vi "BBO.vi"() -> ()   [LabVIEW 2014]
doc: "The myRIO Project template acquires acceleration data from the onboard accelerometer and displays the changes of acceleration values in a waveform chart."
uses:
  <vilib>/vision/driver/NI_Vision_Acquisition_Software.lvlib
  <vilib>/vision/NI_Vision_Development_Module.lvlib
panel:
  in  "배경색ROI밑 자름":dbl=15.0
  in  "위":dbl=60.0
  in  "오른쪽":dbl=60.0
  in  "왼쪽":dbl=40.0
  in  "카메라 X부호":dbl=1.0
  in  "카메라 X":dbl=18.0
  in  "Select Servo 2":string(combo)="Servo 2"
  in  "Threshold Color Mode 3":enum32{"RGB", "HSL"}(radio)=enum."HSL"
  in  "Red or Hue 5":cluster{i32, i32}(slide)={0, 255} scale=0.0..255.0
  in  "Green or Saturation 5":cluster{i32, i32}(slide)={0, 35} scale=0.0..255.0
  in  "Blue or Luminance 5":cluster{i32, i32}(slide)={0, 75} scale=0.0..255.0
  out "볼링핀을찾았는가":bool
  in  "화면전환":bool=TRUE
  out "Image 3":T1(plugin-control)
  in  "공 굴릴 범위":dbl=10.0
  in  "작게 움직이는 범위":dbl=500.0
  in  "탭컨트롤":dbl
  in  "탭 컨트롤":enum32{"볼링핀 0", "녹색핀 1"}(tab)
  in  "Blue or Luminance":cluster{i32, i32}(slide)={90, 255} scale=0.0..255.0
  in  "Green or Saturation":cluster{i32, i32}(slide)={0, 90} scale=0.0..255.0
  in  "Red or Hue":cluster{i32, i32}(slide)={0, 255} scale=0.0..255.0
  in  "Blue or Luminance 3":cluster{i32, i32}(slide)={60, 255} scale=0.0..255.0
  in  "Green or Saturation 3":cluster{i32, i32}(slide)={35, 255} scale=0.0..255.0
  in  "Red or Hue 3":cluster{i32, i32}(slide)={50, 130} scale=0.0..255.0
  in  "좌우모터":i16=25
  in  "Number of Erosion":i32=2
  in  "Threshold Color Mode":enum32{"RGB", "HSL"}(radio)=enum."HSL"
  out "Image 2":T1(plugin-control)
  out "Image":T1(plugin-control)
  in  "Camera Name":refnum<k21>="cam1" caption="IMAQdx Session"
  # "Control Motor"
  # "Read Encoder"
  # "배경색(검은색) 색조"
  # "255"
  # "25"
  # "채도"
  # "HSL : 색조 채도 광도"
  # "35"
  # "광도"
  # "75"
  # "1일때 + 0일때 -"
  # "흰색 : 0/255"
  # "흰색 : 0~90"
  # "흰색 : 90~255"
  # "녹색 : 50/130"
  # "녹색 : 35/255"
  # "녹색 : 60/255"
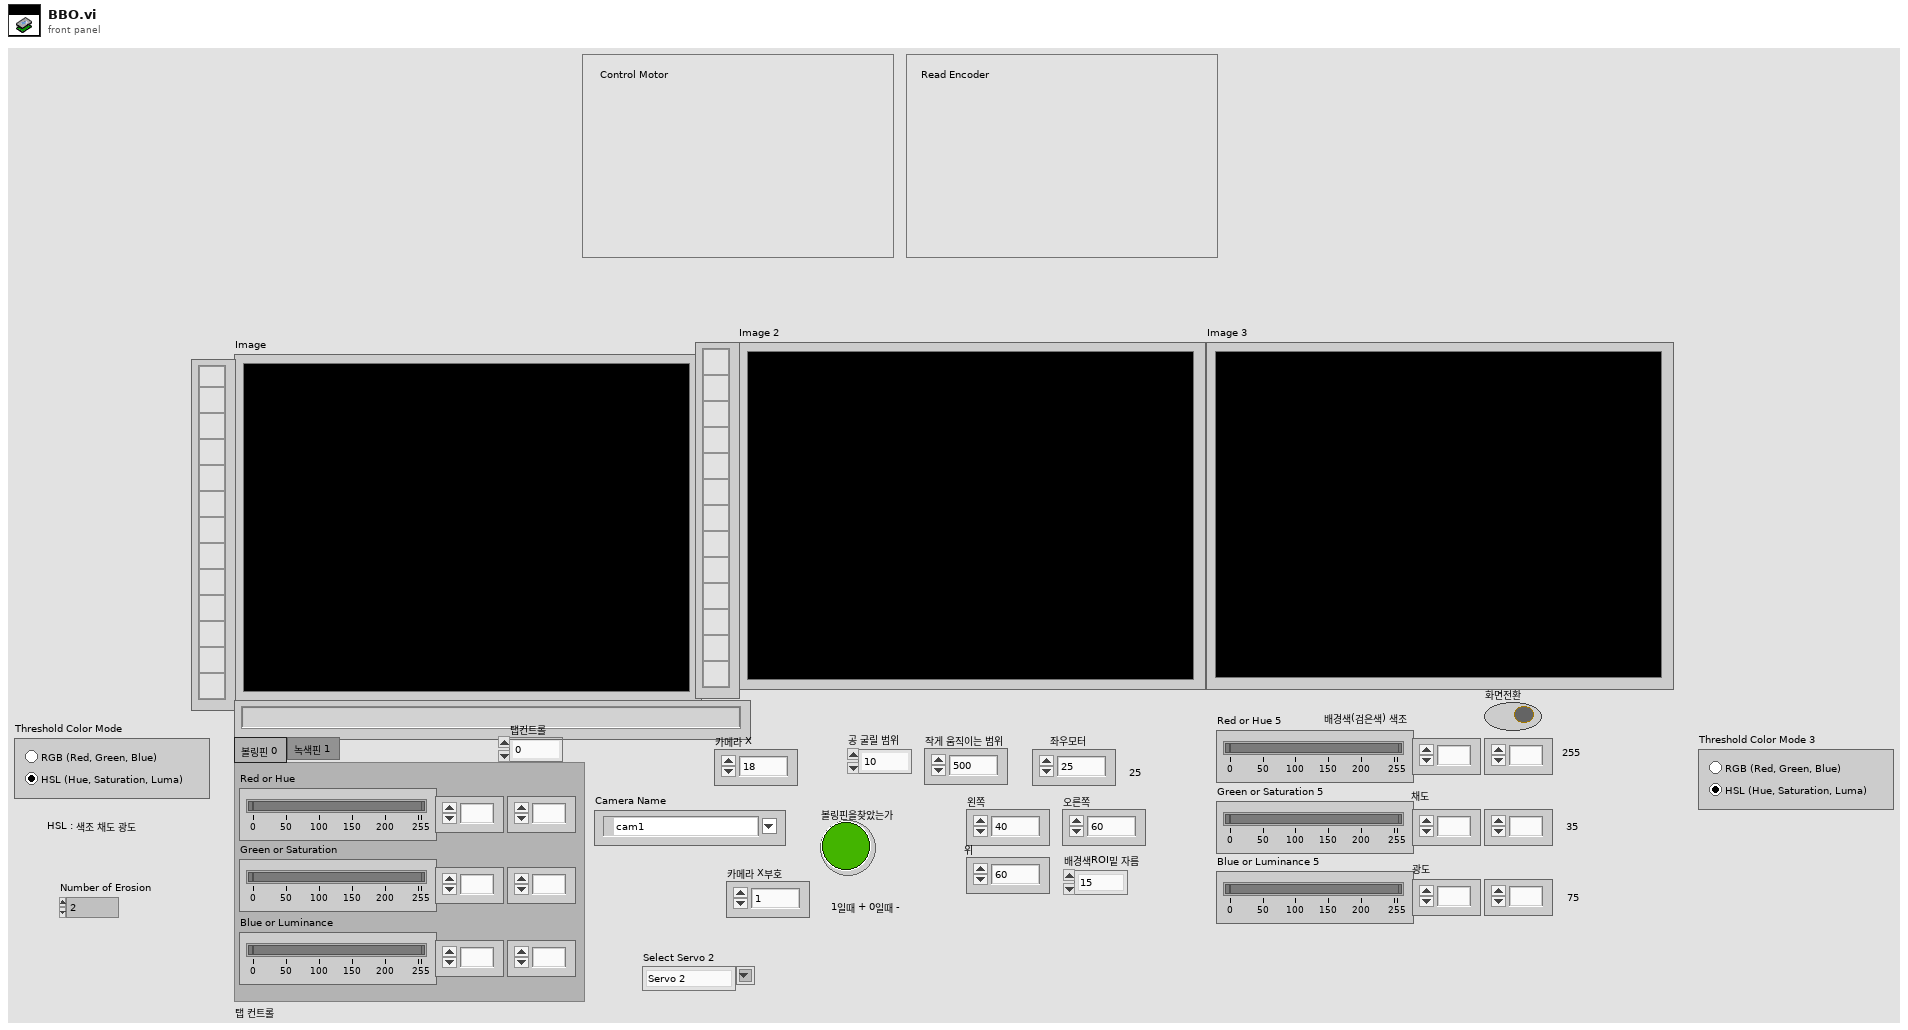
[diagram p1: front panel]
types:
  T1 = typedef "IMAQ Image.ctl" = refnum<image>
  T2 = typedef "IMAQ Rectangle" = cluster{"Left":i32, "Top":i32, "Right":i32, "Bottom":i32, "Rotation":dbl}
  T3 = typedef "Image Type" = u32
  T4 = typedef "IMAQdx.ctl" = refnum<k21>
  T5 = cluster{"Area":dbl, "Number of Holes":dbl, "Bounding Rect":cluster{"Left":dbl, "Top":dbl, "Right":dbl, "Bottom":dbl}, "Center of Mass":cluster{"X":dbl, "Y":dbl}, "Orientation":dbl, "Dimensions":cluster{"Width":dbl, "Height":dbl}}[]
  T6 = cluster{"Area":dbl, "Number of Holes":dbl, "Bounding Rect":cluster{"Left":dbl, "Top":dbl, "Right":dbl, "Bottom":dbl}, "Center of Mass":cluster{"X":dbl, "Y":dbl}, "Orientation":dbl, "Dimensions":cluster{"Width":dbl, "Height":dbl}}
  T7 = cluster{"Left":dbl, "Top":dbl, "Right":dbl, "Bottom":dbl}
  T8 = typedef "ROI Descriptor" = cluster{"Global Rectangle":i32[], "Contours":cluster{"ID":enum32{"External", "Internal"}, "Type":u32, "Coordinates":i32[]}[]}
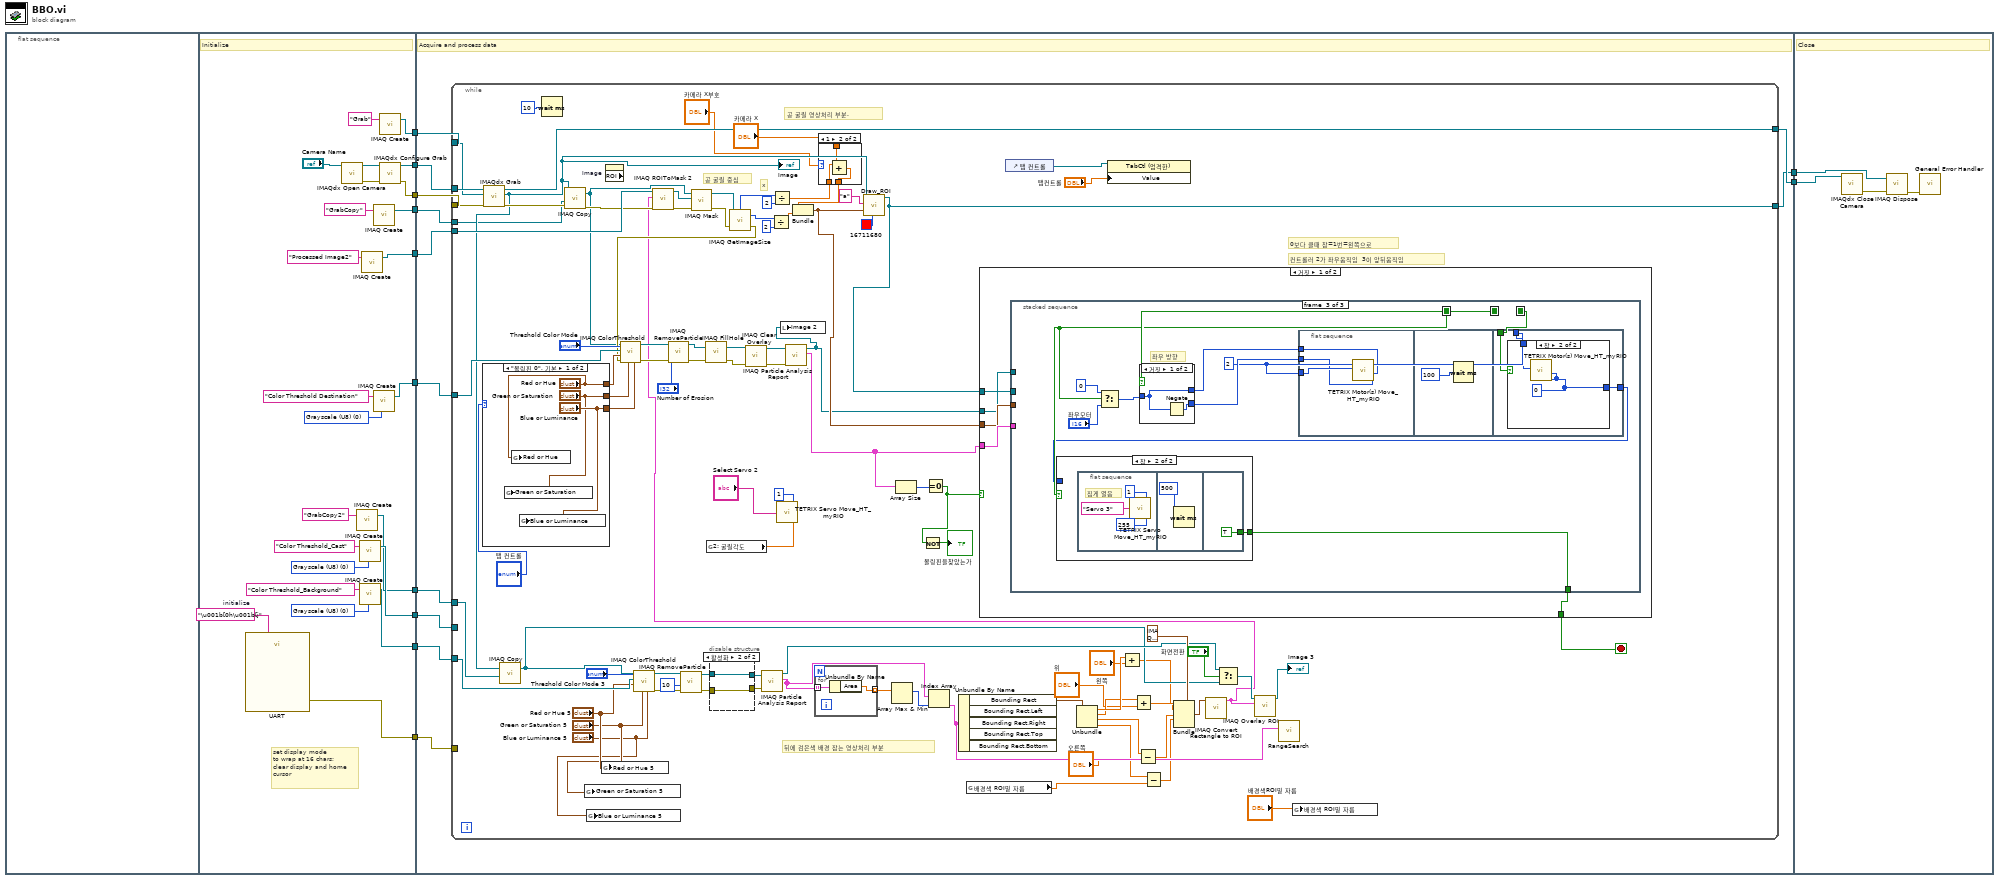
[diagram p0: block diagram]
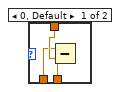
[diagram p2: hidden frame]
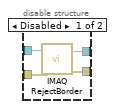
[diagram p3: hidden frame]
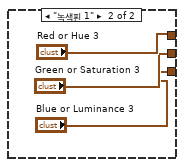
[diagram p4: hidden frame]
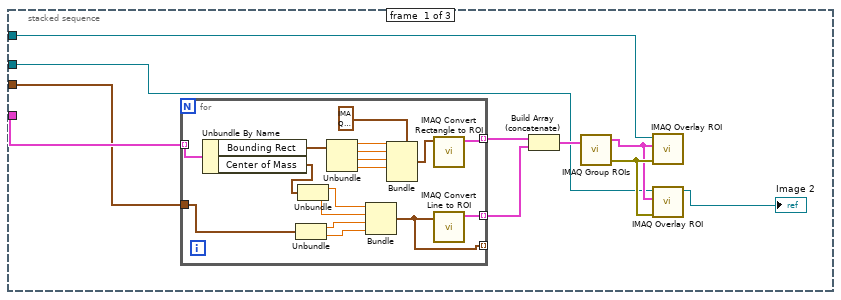
[diagram p5: hidden frame]
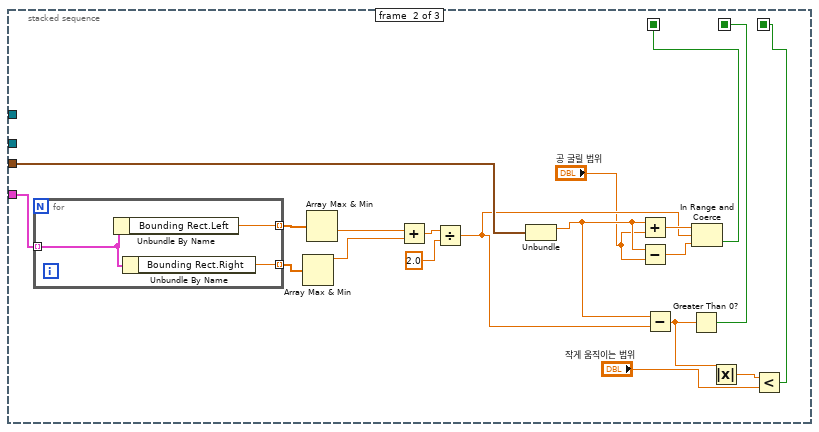
[diagram p6: hidden frame]
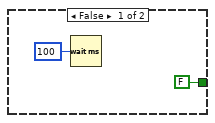
[diagram p7: hidden frame]
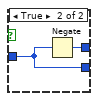
[diagram p9: hidden frame]
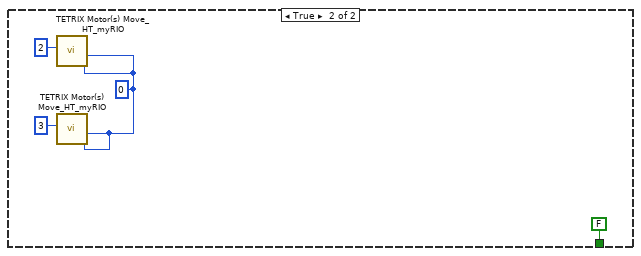
[diagram p10: hidden frame]
diagram:
  n1 = flat-sequence {
    tunnel: [w32] -> w12
    tunnel: [w31] -> w11
    tunnel: [w30] -> w10
    tunnel: [w28] -> w9
    tunnel: [w26] -> w8
    tunnel: [w25] -> w7
    tunnel: [w22] -> w6
    tunnel: [w18] -> w5
    tunnel: [w15] -> w4
    tunnel: [w13] -> w3
    tunnel: w12 -> [w48]
    tunnel: w11 -> [w47]
    tunnel: w10 -> [w46]
    tunnel: [w42] -> w2
    tunnel: [w45] -> w1
    tunnel: w9 -> [w44]
    tunnel: w8 -> [w43]
    tunnel: w7 -> [w37]
    tunnel: w6 -> [w41]
    tunnel: w5 -> [w40]
    tunnel: w4 -> [w39]
    tunnel: w3 -> [w38]
    tunnel: w2 -> [w254]
    tunnel: w1 -> [w253]
    frame #0 {
    }
    frame #1 {
      w16 = T3 0 items=["Grayscale (U8)", "Grayscale (I16)", "Grayscale (SGL)", "Complex (CSG)", "RGB (U32)", "HSL (U32)", "RGB (U64)", "Grayscale (U16)"] ("Image Type")
      w19 = T3 0 items=["Grayscale (U8)", "Grayscale (I16)", "Grayscale (SGL)", "Complex (CSG)", "RGB (U32)", "HSL (U32)", "RGB (U64)", "Grayscale (U16)"] ("Image Type")
      w21 = "\u001b[0h\u001b[j"  # initialize
      w24 = T3 0 items=["Grayscale (U8)", "Grayscale (I16)", "Grayscale (SGL)", "Complex (CSG)", "RGB (U32)", "HSL (U32)", "RGB (U64)", "Grayscale (U16)"] ("Image Type")
      # "set display mode\nto wrap at 16 chars;\nclear display and home\ncursor"
      # "Initialize"
      n2 = call "UART"("Characters to Write"=w21) -> ("error out"=w25:errorcluster)  [unwired: 25 in, 1 out]
      n3 = call <vilib>:"IMAQdx Open Camera.vi"("Session In"="Camera Name") -> ("error out"=w36:errorcluster, "Session Out"=w35:T4)  [unwired: 2 in, 7 out]
      n4 = call "IMAQ Create"("Image Name"="GrabCopy2") -> ("New Image"=w13:T1)  [unwired: 3 in, 2 out]
      n5 = call "IMAQ Create"("Image Name"="Color Threshold_Cast", "Image Type"=w16) -> ("New Image"=w15:T1)  [unwired: 3 in, 1 out]
      n6 = call "IMAQ Create"("Image Name"="Color Threshold_Background", "Image Type"=w19) -> ("New Image"=w18:T1)  [unwired: 3 in, 1 out]
      n7 = call "IMAQ Create"("Image Name"="Processed Image2") -> ("New Image"=w28:T1)  [unwired: 3 in, 2 out]
      n8 = call "IMAQ Create"("Image Name"="Color Threshold Destination", "Image Type"=w24) -> ("New Image"=w22:T1)  [unwired: 3 in, 1 out]
      n9 = call "IMAQ Create"("Image Name"="GrabCopy") -> ("New Image"=w26:T1)  [unwired: 3 in, 2 out]
      n10 = call "IMAQ Create"("Image Name"="Grab") -> ("New Image"=w32:T1)  [unwired: 3 in, 2 out]
      n11 = call <vilib>:"IMAQdx Configure Grab.vi"("error in"=w36, "Session In"=w35) -> ("error out"=w30:errorcluster, "Session Out"=w31:T4)  [unwired: 8 out]
    }
    frame #2 {
      # "Acquire and process data"
      n12 = while {
        tunnel: [w139] -> w45
        tunnel: w46 -> [w141]
        tunnel: w47 -> [w142]
        tunnel: w48 -> [w140]
        tunnel: w44 -> [w137]
        tunnel: w43 -> [w76]
        tunnel: [w106] -> w42
        tunnel: w37 -> [_]
        tunnel: w41 -> [w124]
        tunnel: w40 -> [w84]
        tunnel: w39 -> [_]
        tunnel: w38 -> [w99]
        stop <- w70 stop-if-true
        # "뒤에 검은색 배경 잡는 영상처리 부분"
        # "공 굴릴 영상처리 부분."
        # "0보다 클때 참=1번=왼쪽으로"
        # "컨트롤러 2가 좌우움직임  3이 앞뒤움직임"
        # "공 굴릴 중심"
        # "x"
        n13 = case shown="\"볼링핀 0\", 기본" "탭 컨트롤" {
          tunnel: ["Blue or Luminance" "Blue or Luminance 3"] -> w122
          tunnel: ["Red or Hue" "Red or Hue 3"] -> w121
          tunnel: ["Green or Saturation" "Green or Saturation 3"] -> w120
          frame "볼링핀 0", Default {
            n14 = global write "글로벌.vi" "Green or Saturation"("Green or Saturation") -> ()
            n15 = global write "글로벌.vi" "Red or Hue"("Red or Hue") -> ()
            n16 = global write "글로벌.vi" "Blue or Luminance"("Blue or Luminance") -> ()
          }
          frame "녹색핀 1" {
          }
        }
        n17 = call <vilib>:"IMAQdx Grab.vi"("error in"=w141, "Image In"=w140, "Session In"=w142) -> ("error out"=w127:errorcluster, "Image Out"=w77:T1, "Session Out"=w139:T4)  [unwired: 1 in, 5 out]
        "Image" <- w77
        n18 = call "IMAQ Copy"("Image Dst"=w99, "Image Src"=w77) -> ("Image Dst Out"=w82:T1)  [unwired: 4 in, 1 out]
        n19 = Wait (ms)(milliseconds to wait=u32 10 ("대기 시간(ms)")) -> ()  [unwired: 1 out]
        n20 = call "IMAQ Copy"("error in (no error)"=w127, "Image Dst"=w76, "Image Src"=w77) -> ("error out"=w126:errorcluster, "Image Dst Out"=w74:T1)  [unwired: 3 in]
        n21 = global write "글로벌.vi" "Green or Saturation 5"("Green or Saturation 5") -> ()
        n22 = global write "글로벌.vi" "Blue or Luminance 5"("Blue or Luminance 5") -> ()
        n23 = global write "글로벌.vi" "Red or Hue 5"("Red or Hue 5") -> ()
        n24 = property on="Image" class="ImageControl" props=["ROI"]() -> ()  [unwired: 2 in, 3 out]
        n25 = call "IMAQ ColorThreshold"("Blue or Luma or Val or Inten Range"="Blue or Luminance 5", "Green or Sat Range"="Green or Saturation 5", "Color Mode"="Threshold Color Mode 3", "Red or Hue Range"="Red or Hue 5", "Image Dst"=w84, "Image Src"=w82) -> ("error out"=w89:errorcluster, "Image Dst Out"=w88:T1)  [unwired: 4 in]
        n26 = call "IMAQ RemoveParticle"("error in (no error)"=w89, "Number of Erosion"=10, "Image Src"=w88) -> ("error out"=w91:errorcluster, "Image Dst Out"=w90:T1)  [unwired: 7 in]
        n27 = global read "글로벌.vi" "2: 굴릴각도"() -> (w63:dbl)
        n28 = disable-structure shown="활성화" {
          disable-tunnel: w90 -> [w152 w154]
          disable-tunnel: w91 -> [w151 w153]
          disable-tunnel: [w150 w154] -> w93
          disable-tunnel: [w149 w153] -> w94
          frame Disabled {
            n29 = call "IMAQ RejectBorder"("error in (no error)"=w151, "Image Src"=w152) -> ("error out"=w149:errorcluster, "Image Dst Out"=w150:T1)  [unwired: 4 in]
          }
          frame Enabled {
          }
        }
        n30 = call "IMAQ Particle Analysis Report"("error in (no error)"=w94, "Image"=w93) -> ("Particle Reports (Pixels)"=w86:T5, "Image Out (duplicate)"=w85:T1)  [unwired: 4 in, 4 out]
        n31 = call <vilib>:"TETRIX Servo Move_HT_myRIO.vi"("Servo Position (0 - 255)"=w63, "Controller Daisy Chain Position (1 - 4)"=u8 1, "Select Servo"="Select Servo 2") -> ()  [unwired: 2 in, 1 out]
        n32 = for {
          tunnel: w86 -> [w156] mode=indexing
          tunnel: [w155] -> w104 mode=indexing
          n33 = Unbundle By Name(w156) -> ("Area"=w155:dbl)
        }
        n34 = Array Max & Min(array=w104) -> (max index (indices)=w103:i32)  [unwired: 3 out]
        n35 = Index Array(array=w86, index=w103) -> (element=w97:T6)
        n36 = Unbundle By Name(w97) -> ("Bounding Rect"=w101:T7)  [unwired: 4 out]
        n37 = global read "글로벌.vi" "배경색 ROI밑 자름"() -> (w69:dbl)
        n38 = control-ref of="탭 컨트롤"() -> (w110:refnum<vi>)
        n39 = Unbundle(w101) -> ("Left"=w58:dbl, "Top"=w51:dbl, "Right"=w54:dbl, "Bottom"=w81:dbl)
        n40 = property class="TabCtl (엄격한)"(reference=w110, "Value"="탭컨트롤") -> ()  [unwired: 1 in, 2 out]
        n41 = Add(x=w58, y="왼쪽") -> (x+y=w57:dbl)
        n42 = Add(x=w51, y="위") -> (x+y=w52:dbl)
        n43 = Subtract(x=w54, y="오른쪽") -> (x-y=w53:dbl)
        n44 = Subtract(x=w81, y=w69) -> (x-y=w80:dbl)
        n45 = Bundle(cluster=T2 {"Left"=0, "Top"=0, "Right"=0, "Bottom"=0, "Rotation"=0.0} ("Rectangle"), "Left"=w57, "Top"=w52, "Right"=w53, "Bottom"=w80) -> (w102:T2)  [unwired: 1 in]
        n46 = call "IMAQ Convert Rectangle to ROI"("Rectangle"=w102) -> ("ROI Descriptor"=w71:T8)  [unwired: 8 in, 1 out]
        n47 = call "IMAQ ROIToMask 2"("error in (no error)"=w126, "ROI Descriptor"=w71, "Image"=w137) -> ("error out"=w136:errorcluster, "Image Out"=w75:T1)  [unwired: 6 in, 1 out]
        n48 = call "IMAQ Mask"("error in (no error)"=w136, "Image Mask"=w75, "Image Src"=w74) -> ("error out"=w125:errorcluster, "Image Dst Out"=w78:T1)  [unwired: 2 in]
        n49 = call "IMAQ GetImageSize"("Image"=w78, "error in (no error)"=w125) -> ("Y Resolution"=w131:i32, "X Resolution"=w134:i32, "error out"=w117:errorcluster)  [unwired: 2 in]
        n50 = call "IMAQ ColorThreshold"("Blue or Luma or Val or Inten Range"=w122, "Green or Sat Range"=w120, "Color Mode"="Threshold Color Mode", "error in (no error)"=w117, "Red or Hue Range"=w121, "Image Dst"=w124, "Image Src"=w74) -> ("error out"=w118:errorcluster, "Image Dst Out"=w83:T1)  [unwired: 3 in]
        n51 = call "IMAQ RemoveParticle"("error in (no error)"=w118, "Number of Erosion"="Number of Erosion", "Image Src"=w83) -> ("error out"=w113:errorcluster, "Image Dst Out"=w114:T1)  [unwired: 7 in]
        n52 = call "IMAQ FillHole"("error in (no error)"=w113, "Image Src"=w114) -> ("error out"=w116:errorcluster, "Image Dst Out"=w115:T1)  [unwired: 4 in]
        n53 = call "IMAQ Clear Overlay"("error in (no error)"=w116, "Image"=w115) -> ("error out"=w135:errorcluster, "Image Out"=w138:T1)  [unwired: 1 in, 7 out]
        n54 = Divide(x=w131, y=2) -> (x/y=w130:dbl)
        n55 = Divide(x=w134, y=2) -> (x/y=w61:dbl)
        n56 = call "IMAQ Particle Analysis Report"("error in (no error)"=w135, "Image"=w138) -> ("Particle Reports (Pixels)"=w79:T5, "Image Out (duplicate)"=w105:T1)  [unwired: 4 in, 4 out]
        n57 = local write "Image 2"(w105) -> ()
        n58 = case shown="1" "카메라 X부호" {
          tunnel: [w143 w148] -> w62
          tunnel: w61 -> [w144 w147]
          tunnel: "카메라 X" -> [w145 w146]
          frame 0, Default {
            n59 = Subtract(x=w144, y=w145) -> (x-y=w143:dbl)
          }
          frame 1 {
            n60 = Add(x=w147, y=w146) -> (x+y=w148:dbl)
          }
        }
        n61 = Bundle(w62, w130) -> (w108:cluster{dbl, dbl})  [unwired: 1 in]
        n62 = call "Draw_ROI.vi"("Color"=u32 16711680, "클러스터"=w108, "Group"="a", "참조 번호 입력"=w77) -> ("참조 번호 출력"=w106:T1)  [unwired: 7 in]
        n63 = Array Size(array=w79) -> (size(s)=w112:i32)
        n64 = Equal To 0?(x=w112) -> (x = 0?=w95:bool)
        n65 = Not(x=w95) -> (.not. x?=→"볼링핀을찾았는가":bool)
        n66 = case shown="거짓" w95 {
          tunnel: w79 -> [w167 _]
          tunnel: w108 -> [w166 _]
          tunnel: w105 -> [w165 _]
          tunnel: w106 -> [w164 _]
          tunnel: [w163 FALSE] -> w70
          frame False {
            n67 = stacked-sequence {
              seq-local: [_ w195 _] -> [_ _ w225]
              seq-local: [_ w201 _] -> [_ _ w227]
              seq-local: [_ w197 _] -> [_ _ w226]
              tunnel: w167 -> [w172 w205 _]
              tunnel: w166 -> [w169 w204 _]
              tunnel: w165 -> [w171 _ _]
              tunnel: w164 -> [w170 _ _]
              tunnel: [_ _ w217] -> w163
              frame #0 {
                n68 = for {
                  tunnel: w172 -> [w194] mode=indexing
                  tunnel: [w186] -> w174 mode=indexing
                  tunnel: w169 -> [w182]
                  tunnel: [w179] -> w176 mode=indexing
                  tunnel: [w178] -> _ mode=indexing
                  n69 = Unbundle By Name(w194) -> ("Bounding Rect"=w192:T7, "Center of Mass"=w185:cluster{"X":dbl, "Y":dbl})
                  n70 = Unbundle(w182) -> (w181:dbl, w180:dbl)
                  n71 = Unbundle(w185) -> ("X"=w184:dbl, "Y"=w183:dbl)
                  n72 = Unbundle(w192) -> ("Left"=w191:dbl, "Top"=w190:dbl, "Right"=w189:dbl, "Bottom"=w188:dbl)
                  n73 = Bundle("X"=w184, "Y"=w183, w181, w180) -> (w178:cluster{"X":dbl, "Y":dbl, dbl, dbl})  [unwired: 1 in]
                  n74 = Bundle(cluster=T2 {"Left"=0, "Top"=0, "Right"=0, "Bottom"=0, "Rotation"=0.0} ("Rectangle"), "Left"=w191, "Top"=w190, "Right"=w189, "Bottom"=w188) -> (w187:T2)  [unwired: 1 in]
                  n75 = call "IMAQ Convert Rectangle to ROI"("Rectangle"=w187) -> ("ROI Descriptor"=w186:T8)  [unwired: 8 in, 1 out]
                  n76 = call "IMAQ Convert Line to ROI"("Line"=w178) -> ("ROI Descriptor"=w179:T8)  [unwired: 8 in, 1 out]
                }
                n77 = Build Array (concatenate)(w174, w176) -> (w175:T8[])
                n78 = call "IMAQ Group ROIs"("ROI Descriptors"=w175) -> ("error out"=w177:errorcluster, "ROI Descriptor out"=w173:T8)  [unwired: 1 in, 2 out]
                n79 = call "IMAQ Overlay ROI"("error in (no error)"=w177, "ROI Descriptor"=w173, "Image"=w170) -> ()  [unwired: 3 in, 6 out]
                n80 = call "IMAQ Overlay ROI"("error in (no error)"=w177, "ROI Descriptor"=w173, "Image"=w171) -> ("Image Out"=→"Image 2":T1)  [unwired: 3 in, 5 out]
              }
              frame #1 {
                n81 = for {
                  tunnel: w205 -> [w216] mode=indexing
                  tunnel: [w215] -> w210 mode=indexing
                  tunnel: [w214] -> w212 mode=indexing
                  n82 = Unbundle By Name(w216) -> ("Bounding Rect.Left"=w215:dbl)
                  n83 = Unbundle By Name(w216) -> ("Bounding Rect.Right"=w214:dbl)
                }
                n84 = Array Max & Min(array=w212) -> (max value=w213:dbl)  [unwired: 3 out]
                n85 = Array Max & Min(array=w210) -> (min value=w211:dbl)  [unwired: 3 out]
                n86 = Add(x=w211, y=w213) -> (x+y=w206:dbl)
                n87 = Divide(x=w206, y=2.0) -> (x/y=w202:dbl)
                n88 = Unbundle(w204) -> (w203:dbl)  [unwired: 1 out]
                n89 = Add(x=w203, y="공 굴릴 범위") -> (x+y=w208:dbl)
                n90 = Subtract(x=w203, y="공 굴릴 범위") -> (x-y=w209:dbl)
                n91 = Subtract(x=w203, y=w202) -> (x-y=w200:dbl)
                n92 = Greater Than 0?(x=w200) -> (x > 0?=w201:bool)
                n93 = In Range and Coerce(upper limit=w208, x=w202, lower limit=w209) -> (In Range?=w195:bool)  [unwired: 1 out]
                n94 = Absolute Value(x=w200) -> (abs(x)=w199:dbl)
                n95 = Less?(x=w199, y="작게 움직이는 범위") -> (x < y?=w197:bool)
              }
              frame #2 {
                w220 = u8 2 ("Controller 2")
                # "좌우 방향"
                n96 = case shown="참" w225 {
                  tunnel: w218 -> [_ _]
                  tunnel: [FALSE w230] -> w217
                  frame False {
                    n97 = Wait (ms)(milliseconds to wait=u32 100 ("대기 시간(ms)")) -> ()  [unwired: 1 out]
                  }
                  frame True {
                    n98 = flat-sequence {
                      tunnel: [TRUE] -> w230
                      frame #0 {
                        # "집게 열음"
                        n99 = call <vilib>:"TETRIX Servo Move_HT_myRIO.vi"("Servo Position (0 - 255)"=u8 255, "Controller Daisy Chain Position (1 - 4)"=u8 1, "Select Servo"="Servo 3") -> ()  [unwired: 2 in, 1 out]
                      }
                      frame #1 {
                        n100 = Wait (ms)(milliseconds to wait=u32 500 ("대기 시간(ms)")) -> ()  [unwired: 1 out]
                      }
                      frame #2 {
                      }
                    }
                  }
                }
                n101 = Select(t=i8 0 ("Motor 2 Power (-100 to 100)\n0 = Stop/Brake\n-128 = Stop/Coast"), s=w225, f="좌우모터") -> (s? t:f=w222:i16)
                n102 = case shown="거짓" w227 {
                  tunnel: [w246 w248] -> w224
                  tunnel: w222 -> [w246 w247]
                  tunnel: [w245 w247] -> w223
                  frame False {
                    n103 = Negate(x=w246) -> (-x=w245:i16)
                  }
                  frame True {
                    n104 = Negate(x=w247) -> (-x=w248:i16)
                  }
                }
                n105 = flat-sequence {
                  tunnel: w220 -> [w238]
                  tunnel: w224 -> [w237]
                  tunnel: w223 -> [w236]
                  tunnel: w220 -> [w242]
                  tunnel: w226 -> [w241]
                  tunnel: [w240] -> w218
                  frame #0 {
                    n106 = call <vilib>:"TETRIX Motor(s) Move_HT_myRIO.vi"("Motor 2 Power (-100 to 100)\n0 = Stop/Brake\n-128 = Stop/Coast"=w236, "Motor 1 Power (-100 to 100)\n0 = Stop/Brake\n-128 = Stop/Coast"=w237, "Controller Daisy Chain Position: 1 - 4"=w238) -> ()  [unwired: 6 in, 1 out]
                  }
                  frame #1 {
                    n107 = Wait (ms)(milliseconds to wait=u32 100 ("대기 시간(ms)")) -> ()  [unwired: 1 out]
                  }
                  frame #2 {
                    n108 = case shown="참" w241 {
                      tunnel: w242 -> [_ w244]
                      tunnel: [_ w243] -> w240
                      frame False {
                      }
                      frame True {
                        w243 = i8 0 ("Motor 2 Power (-100 to 100)\n0 = Stop/Brake\n-128 = Stop/Coast")
                        n109 = call <vilib>:"TETRIX Motor(s) Move_HT_myRIO.vi"("Motor 2 Power (-100 to 100)\n0 = Stop/Brake\n-128 = Stop/Coast"=w243, "Motor 1 Power (-100 to 100)\n0 = Stop/Brake\n-128 = Stop/Coast"=w243, "Controller Daisy Chain Position: 1 - 4"=w244) -> ()  [unwired: 6 in, 1 out]
                      }
                    }
                  }
                }
              }
            }
          }
          frame True {
            w250 = 0
            n110 = call <vilib>:"TETRIX Motor(s) Move_HT_myRIO.vi"("Motor 2 Power (-100 to 100)\n0 = Stop/Brake\n-128 = Stop/Coast"=w250, "Motor 1 Power (-100 to 100)\n0 = Stop/Brake\n-128 = Stop/Coast"=w250, "Controller Daisy Chain Position: 1 - 4"=u8 2) -> ()  [unwired: 6 in, 1 out]
            n111 = call <vilib>:"TETRIX Motor(s) Move_HT_myRIO.vi"("Motor 2 Power (-100 to 100)\n0 = Stop/Brake\n-128 = Stop/Coast"=w250, "Motor 1 Power (-100 to 100)\n0 = Stop/Brake\n-128 = Stop/Coast"=w250, "Controller Daisy Chain Position: 1 - 4"=u8 3) -> ()  [unwired: 6 in, 1 out]
          }
        }
        n112 = Select(t=w85, s="화면전환", f=w82) -> (s? t:f=w73:T1)
        n113 = call "IMAQ Overlay ROI"("ROI Descriptor"=w71, "Image"=w73) -> ("Image Out"=→"Image 3":T1)  [unwired: 4 in, 5 out]
        n114 = call "RangeSearch.vi"("Particle Report"=w97) -> ()  [unwired: 10 in, 1 out]
        n115 = global write "글로벌.vi" "배경색 ROI밑 자름"("배경색ROI밑 자름") -> ()
      }
    }
    frame #3 {
      # "Close"
      n116 = call <vilib>:"IMAQdx Close Camera.vi"("Session In"=w253) -> ("error out"=w256:errorcluster)  [unwired: 1 in, 9 out]
      n117 = call "IMAQ Dispose"("Image"=w254, "error in (no error)"=w256) -> ("error out"=w255:errorcluster)  [unwired: 4 in]
      n118 = call <vilib>:"General Error Handler.vi"("error in (no error)"=w255) -> ()  [unwired: 2 in, 13 out]
    }
  }
